vi "De-Initialize.vi"(8 "error in (no error)":errorcluster, 11 "DAQmx Digitizer in":refnum<class "DAQmx Digitizer.lvclass">) -> (0 "error out":errorcluster, 3 "DAQmx Digitizer out":refnum<class "DAQmx Digitizer.lvclass">)   [LabVIEW 2021, in "DAQmx Digitizer.lvclass"]
uses:
  DAQmx Digitizer.lvclass
  DAQmx Digitizer.lvclass/DAQmx Digitizer.ctl
  Instruments/Pulse Driver/Lockin Digitizer Driver/Lockin Digitizer Driver.lvclass
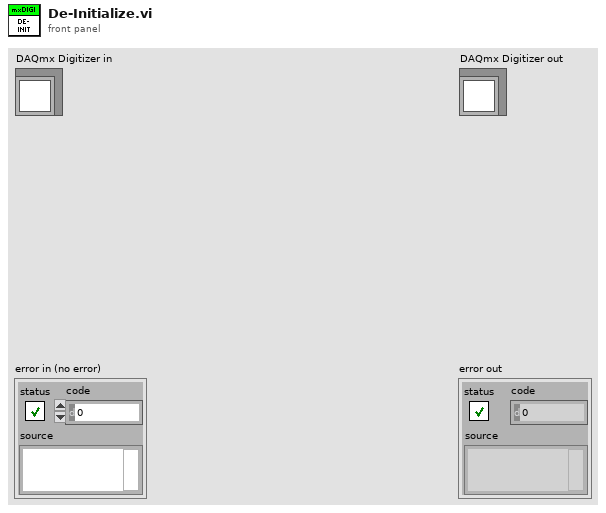
[diagram p1: front panel]
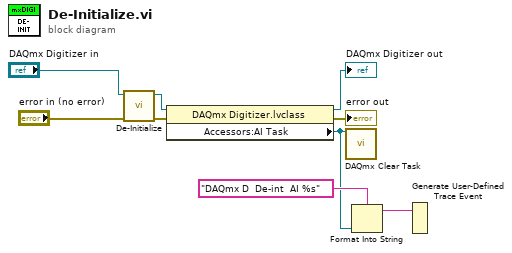
[diagram p0: block diagram]
diagram:
  n1 = call-parent "De-Initialize.vi"("error in (no error)"="error in (no error)", "Instrument Driver in"="DAQmx Digitizer in") -> ("error out"=w3:errorcluster, "Instrument Driver out"=w5:refnum<class "DAQmx Digitizer.lvclass">)  [unwired: 8 in]
  n2 = property class="DAQmx Digitizer.lvclass"(reference=w5, error in=w3) -> (reference out=→"DAQmx Digitizer out":refnum<class "DAQmx Digitizer.lvclass">, error out=→"error out":errorcluster, "Accessors:AI Task"=w1:refnum<k21>)
  n3 = call <vilib>:"DAQmx Clear Task.vi"("task in"=w1) -> ()  [unwired: 14 in, 1 out]
  n4 = Format Into String(format string="DAQmx D  De-int  AI %s" ("string"), w1) -> (resulting string=w7:string)  [unwired: 2 in, 1 out]
  n5 = Generate User-Defined Trace Event(2:w7) -> ()  [unwired: 1 in]
